vi "Read Channels.vi"(8 "error in (no error)":errorcluster, 11 "CIF_UI in":refnum<class "CIF_UI.lvclass">) -> (0 "error out":errorcluster, 2 "Channels":T1[](array[typedef]), 3 "CIF_UI out":refnum<class "CIF_UI.lvclass">)   [LabVIEW 2021, in "CIF_UI.lvclass"]
uses:
  CIF_UI.lvclass
  CIFCore/Grpc/CIFCoreChannel_client/RPC Messages/cif_management_common_Channel.ctl
  CIFCore/Grpc/CIFCoreChannel_client/RPC Messages/cif_management_common_ChannelDirection.ctl
  CIFCore/Grpc/CIFCoreChannel_client/RPC Messages/cif_management_common_ChannelPattern.ctl
  CIF_UI.lvclass/CIF_UI.ctl
  CIFCore/Grpc/CIFCoreChannel_client/CIFCoreChannel_client.lvlib
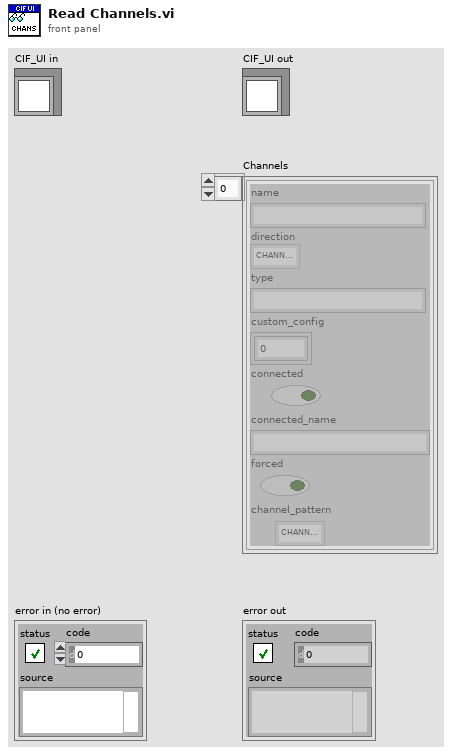
[diagram p1: front panel]
types:
  T1 = typedef "CIFCoreChannel_client.lvlib/cif_management_common_Channel.ctl" = cluster{"name":string, "direction":T2, "type":string, "custom_config":u8[], "connected":bool, "connected_name":string, "forced":bool, "channel_pattern":T3}
  T2 = typedef "CIFCoreChannel_client.lvlib/cif_management_common_ChannelDirection.ctl" = enum32{"CHANNELDIRECTION_UNKNOWN", "CHANNELDIRECTION_PUBLISHER", "CHANNELDIRECTION_SUBSCRIBER"}
  T3 = typedef "CIFCoreChannel_client.lvlib/cif_management_common_ChannelPattern.ctl" = enum32{"CHANNELPATTERN_UNKNOWN", "CHANNELPATTERN_TAG", "CHANNELPATTERN_FIFO", "CHANNELPATTERN_MULTIFIFO", "CHANNELPATTERN_BACKPRESSUREFIFO"}
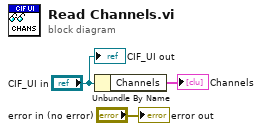
[diagram p0: block diagram]
diagram:
  n1 = Unbundle By Name("CIF_UI in") -> ("Channels"=→"Channels":T1[])
  "error out" <- "error in (no error)"
  "CIF_UI out" <- "CIF_UI in"
